vi "ma_Process DC for N Blocks.vi"(6 "reset":bool, 7 "window for DC":T2(ring)=enum."Hanning", 8 "time signal data (samples)":dbl[][](array[numeric])=[[1.0, 1.0]] format="%0.2p", 10 "averaging type":enum16{"Linear", "Exponential"}(ring), 11 "state info":T1 {"buffer" format="%0.2f"; "timestamp" format="%<%.4X>T"; "dt history" format="%0.2f"; "t0 history" format="%<%I:%M:%S%4u %p>T"; "exp TC (samples)" format="%0.2f"; "RMS history" format="%0.2f"; "DC history" format="%0.2f"}) -> (2 "DC value data":dbl[](array[numeric]) format="%0.6p", 3 "state info":T1 {"buffer" format="%0.2f"; "timestamp" format="%<%.4X>T"; "dt history" format="%0.2f"; "t0 history" format="%<%I:%M:%S%4u %p>T"; "exp TC (samples)" format="%0.2f"; "RMS history" format="%0.2f"; "DC history" format="%0.2f"})   [LabVIEW 2020, in "NI_MAPro.lvlib"]
uses:
  NI_MAPro.lvlib
  NI_AALBase.lvlib
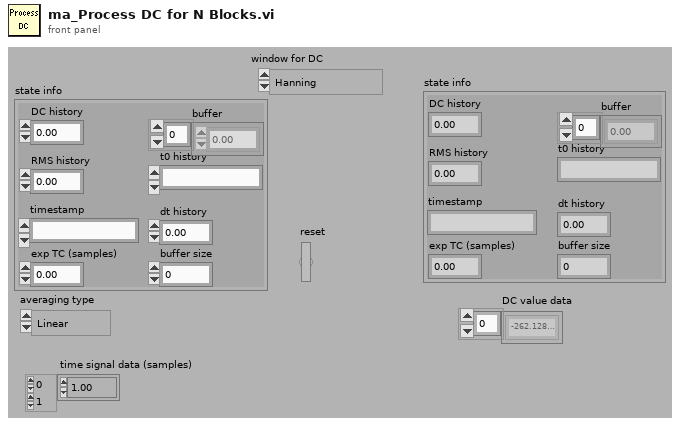
[diagram p1: front panel]
types:
  T1 = cluster{"DC history":dbl, "RMS history":dbl, "exp TC (samples)":dbl, "buffer size":i32, "t0 history":timestamp, "dt history":dbl, "timestamp":timestamp, "buffer":dbl[]}
  T2 = enum16{"Rectangular (none)", "Hanning", "Low side lobe"}
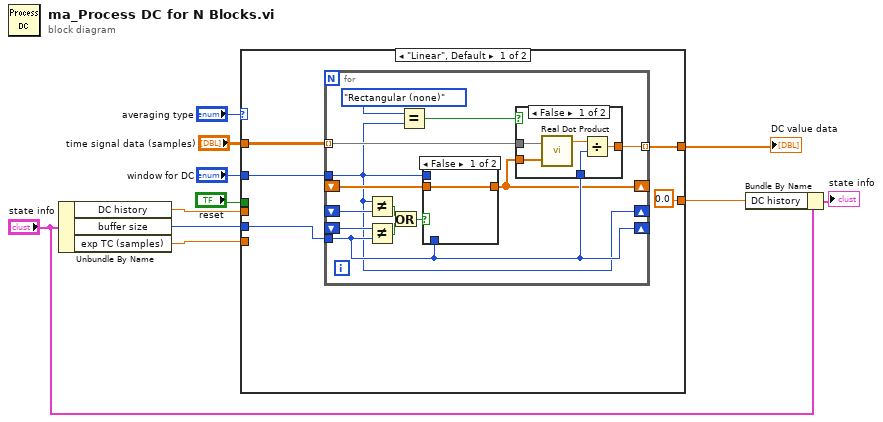
[diagram p0: block diagram]
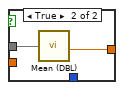
[diagram p2: hidden frame]
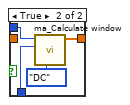
[diagram p3: hidden frame]
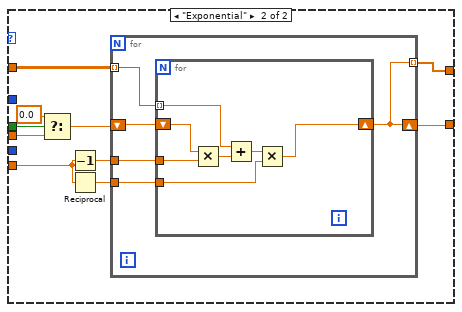
[diagram p4: hidden frame]
diagram:
  n1 = Unbundle By Name("state info") -> ("DC history"=w8:dbl, "buffer size"=w5:i32, "exp TC (samples)"=w7:dbl)
  n2 = case shown="\"Linear\", Default" "averaging type" {
    tunnel: w5 -> [w15 _]
    tunnel: "time signal data (samples)" -> [w14 w51]
    tunnel: [w16 w47] -> w6
    tunnel: w7 -> [_ w49]
    tunnel: [0.0 w46] -> w2
    tunnel: "window for DC" -> [w12 _]
    tunnel: "reset" -> [_ w44]
    tunnel: w8 -> [_ w43]
    frame "Linear", Default {
      n3 = for {
        tunnel: [w29] -> w16 mode=indexing
        tunnel: w15 -> [w27]
        tunnel: w14 -> [w28] mode=indexing
        shift-right: [w17] -> _
        shift-left: _ -> [w25]
        shift-right: [w27] -> _
        shift-left: _ -> [w24]
        shift-right: [w26] -> _
        shift-left: _ -> [w23]
        tunnel: w12 -> [w17]
        n4 = Not Equal?(x=w17, y=w25) -> (x != y?=w22:bool)
        n5 = Not Equal?(x=w24, y=w27) -> (x != y?=w21:bool)
        n6 = Or(x=w22, y=w21) -> (x .or. y?=w20:bool)
        n7 = Equal?(x=T2."Rectangular (none)", y=w17) -> (x = y?=w18:bool)
        n8 = case shown="False" w20 {
          tunnel: w17 -> [_ w41]
          tunnel: w27 -> [_ w40]
          tunnel: [w37 w38] -> w26
          tunnel: w23 -> [w37 _]
          frame False {
          }
          frame True {
            n9 = call "ma_Calculate window.vi"("scaled for"=enum16{"DC", "RMS"}."DC", "array size"=w40, "window"=w41) -> ("Window data"=w38:dbl[])  [unwired: 8 in]
          }
        }
        n10 = case shown="False" w18 {
          tunnel: w28 -> [w34 w36]
          tunnel: [w33 w35] -> w29
          tunnel: w26 -> [w32 _]
          tunnel: w27 -> [w31 _]
          frame False {
            n11 = call "Real Dot Product.vi"("Y Vector"=w32, "X Vector"=w34) -> ("X * Y"=w30:dbl)  [unwired: 1 out]
            n12 = Divide(x=w30, y=w31) -> (x/y=w33:dbl)
          }
          frame True {
            n13 = call "Mean (DBL).vi"("X"=w36) -> ("mean"=w35:dbl)  [unwired: 1 out]
          }
        }
      }
    }
    frame "Exponential" {
      n14 = Select(t=0.0, s=w44, f=w43) -> (s? t:f=w45:dbl)
      n15 = Decrement(x=w49) -> (x-1=w50:dbl)
      n16 = Reciprocal(x=w49) -> (1/x=w48:dbl)
      n17 = for {
        tunnel: w51 -> [w56] mode=indexing
        tunnel: w50 -> [w55]
        tunnel: [w52] -> w47 mode=indexing
        tunnel: w48 -> [w54]
        shift-right: [w52] -> w46
        shift-left: w45 -> [w53]
        n18 = for {
          tunnel: w56 -> [w58] mode=indexing
          shift-right: [w57] -> w52
          shift-left: w53 -> [w62]
          tunnel: w55 -> [w63]
          tunnel: w54 -> [w59]
          n19 = Multiply(x=w62, y=w63) -> (x*y=w61:dbl)
          n20 = Add(x=w58, y=w61) -> (x+y=w60:dbl)
          n21 = Multiply(x=w60, y=w59) -> (x*y=w57:dbl)
        }
      }
    }
  }
  "DC value data" <- w6
  n22 = Bundle By Name(cluster="state info", "DC history"=w2) -> (→"state info":T1)
